vi "GE 5565PIORC.DMA.Block.Allocate.vi"(8 "error in (no error)":errorcluster, 10 "size in bytes":u32, 11 "GE 5565PIORC in":refnum<class "GE 5565PIORC.lvclass">) -> (0 "error out":errorcluster, 2 "Block Descriptor":T1 {"descriptor params"."data ptr (lower)" format="%.0x"; "descriptor params"."data ptr (upper)" format="%.0x"; "descriptor params"."data size" format="%.0x"; "descriptor params"."next descriptor ptr" format="%.0x"; "descriptor size" format="%08x"; "descriptor ptr (RFM)" format="%08x"; "descriptor ptr (VISA)" format="%08x"}, 3 "GE 5565PIORC out":refnum<class "GE 5565PIORC.lvclass">)   [LabVIEW 2024, in "GE 5565PIORC.lvclass"]
doc: "Allocates a new block of memory of length <B>size in bytes</B> using VISA MEMACC."
uses:
  GE 5565PIORC.lvclass
  Typedefs/GE 5565PIORC.Typedef.DMA Block Descriptor.ctl
  Typedefs/GE 5565PIORC.Typedef.DMA Block Descriptor Params.ctl
  GE 5565PIORC.lvclass/GE 5565PIORC.ctl
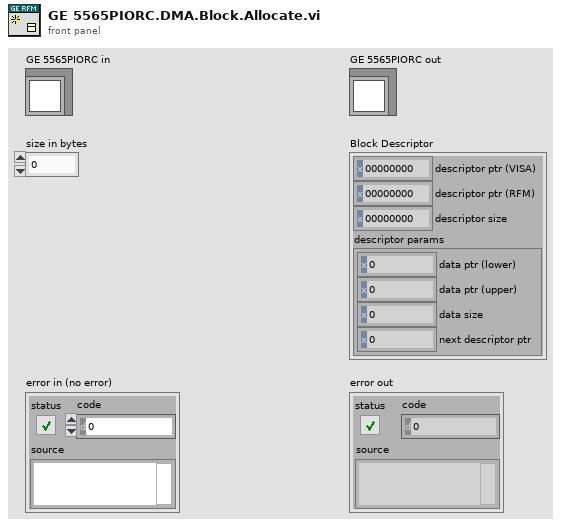
[diagram p1: front panel]
types:
  T1 = typedef "GE 5565PIORC.lvclass/GE 5565PIORC.Typedef.DMA Block Descriptor.ctl" = cluster{"descriptor ptr (VISA)":u32, "descriptor ptr (RFM)":u32, "descriptor size":u32, "descriptor params":T2}
  T2 = typedef "GE 5565PIORC.lvclass/GE 5565PIORC.Typedef.DMA Block Descriptor Params.ctl" = cluster{"data ptr (lower)":u32, "data ptr (upper)":u32, "data size":u32, "next descriptor ptr":u32}
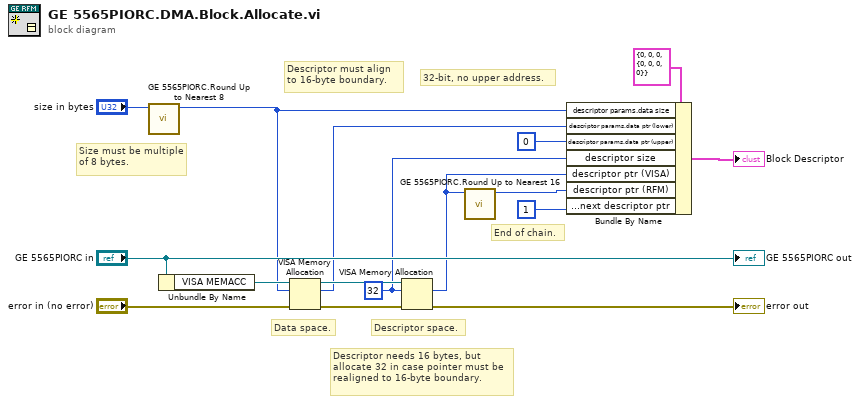
[diagram p0: block diagram]
diagram:
  w11 = u32 32 ("size")
  # "Descriptor needs 16 bytes, but allocate 32 in case pointer must be realigned to 16-byte boundary."
  # "Descriptor must align to 16-byte boundary."
  # "Descriptor space."
  # "Data space."
  # "32-bit, no upper address."
  # "End of chain."
  # "Size must be multiple of 8 bytes."
  n1 = call "GE 5565PIORC.Round Up to Nearest 8.vi"("value"="size in bytes") -> ("aligned value"=w4:u32)  [unwired: 10 in]
  n2 = Unbundle By Name("GE 5565PIORC in") -> ("VISA MEMACC"=w9:refnum<visa-resource-name>)
  n3 = VISA Memory Allocation(8:"error in (no error)", 10:w4, 11:w9) -> (0:w14:errorcluster, 2:w6:u32, 3:w13:refnum<visa-resource-name>)
  n4 = VISA Memory Allocation(8:w14, 10:w11, 11:w13) -> (0:→"error out":errorcluster, 2:w3:u32)  [unwired: 1 out]
  n5 = call "GE 5565PIORC.Round Up to Nearest 16.vi"("value"=w3) -> ("aligned value"=w2:u32)  [unwired: 10 in]
  n6 = Bundle By Name(cluster=T1 {"descriptor ptr (VISA)"=0, "descriptor ptr (RFM)"=0, "descriptor size"=0, "descriptor params"={"data ptr (lower)"=0, "data ptr (upper)"=0, "data size"=0, "next descriptor ptr"=0}} ("Block Descriptor"), "descriptor params.data size"=w4, "descriptor params.data ptr (lower)"=w6, "descriptor params.data ptr (upper)"=u32 0 ("next block pointer"), "descriptor size"=w11, "descriptor ptr (VISA)"=w3, "descriptor ptr (RFM)"=w2, "descriptor params.next descriptor ptr"=u32 1 ("next block pointer")) -> (→"Block Descriptor":T1)
  "GE 5565PIORC out" <- "GE 5565PIORC in"
